vi "delay_time_control.vi"(1 "Higher limit":dbl=100.0 min=0.0 max=100.0 format="%#_13g", 2 "values in":cluster{"delay_time":string}) -> (6 "delay time":dbl)   [LabVIEW 2015]
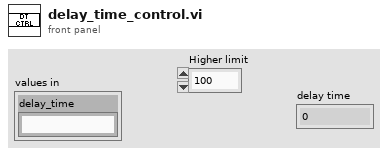
[diagram p1: front panel]
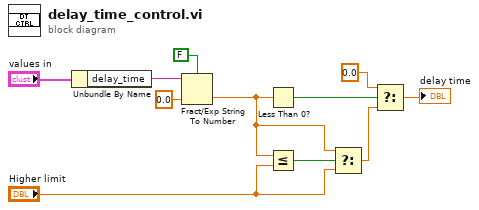
[diagram p0: block diagram]
diagram:
  n1 = Unbundle By Name("values in") -> ("delay_time"=w10:string)
  n2 = Fract/Exp String To Number(use system decimal point (T)=FALSE, string=w10, default (0 dbl)=0.0 ("default (0 I32)")) -> (number=w2:dbl)  [unwired: 1 in, 1 out]
  n3 = Less Than 0?(x=w2) -> (x < 0?=w3:bool)
  n4 = Less Or Equal?(x=w2, y="Higher limit") -> (x <= y?=w6:bool)
  n5 = Select(t=w2, s=w6, f="Higher limit") -> (s? t:f=w5:dbl)
  n6 = Select(t=0.0, s=w3, f=w5) -> (s? t:f=→"delay time":dbl)
